vi "LMS_SetupStream.vi"(8 "error in (no error)":errorcluster, 10 "stream_In":T1, 11 "device_In":i64) -> (0 "error out":errorcluster, 1 "steam_Out":T1, 3 "device_Out":i64)   [LabVIEW 2013, in "LMS_LV_Drv.lvlib"]
uses:
  LMS_LV_Drv.lvlib
  Stream_ctl.ctl
  LimeSuite.dll
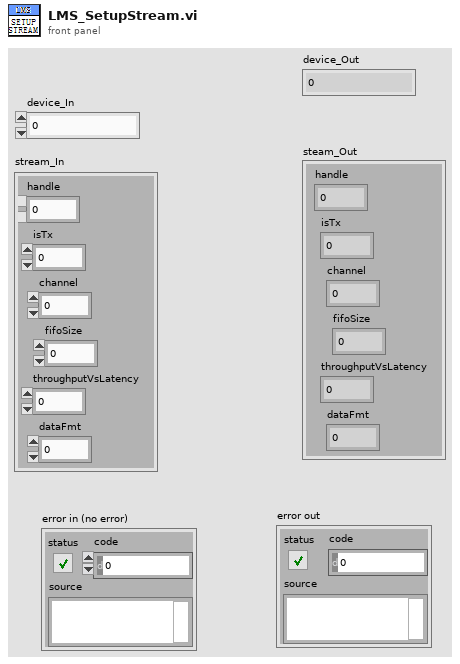
[diagram p1: front panel]
types:
  T1 = typedef "Stream_ctl.ctl" = cluster{"handle":u64, "isTx":u8, "channel":u32, "fifoSize":u32, "throughputVsLatency":dbl, "dataFmt":u32}
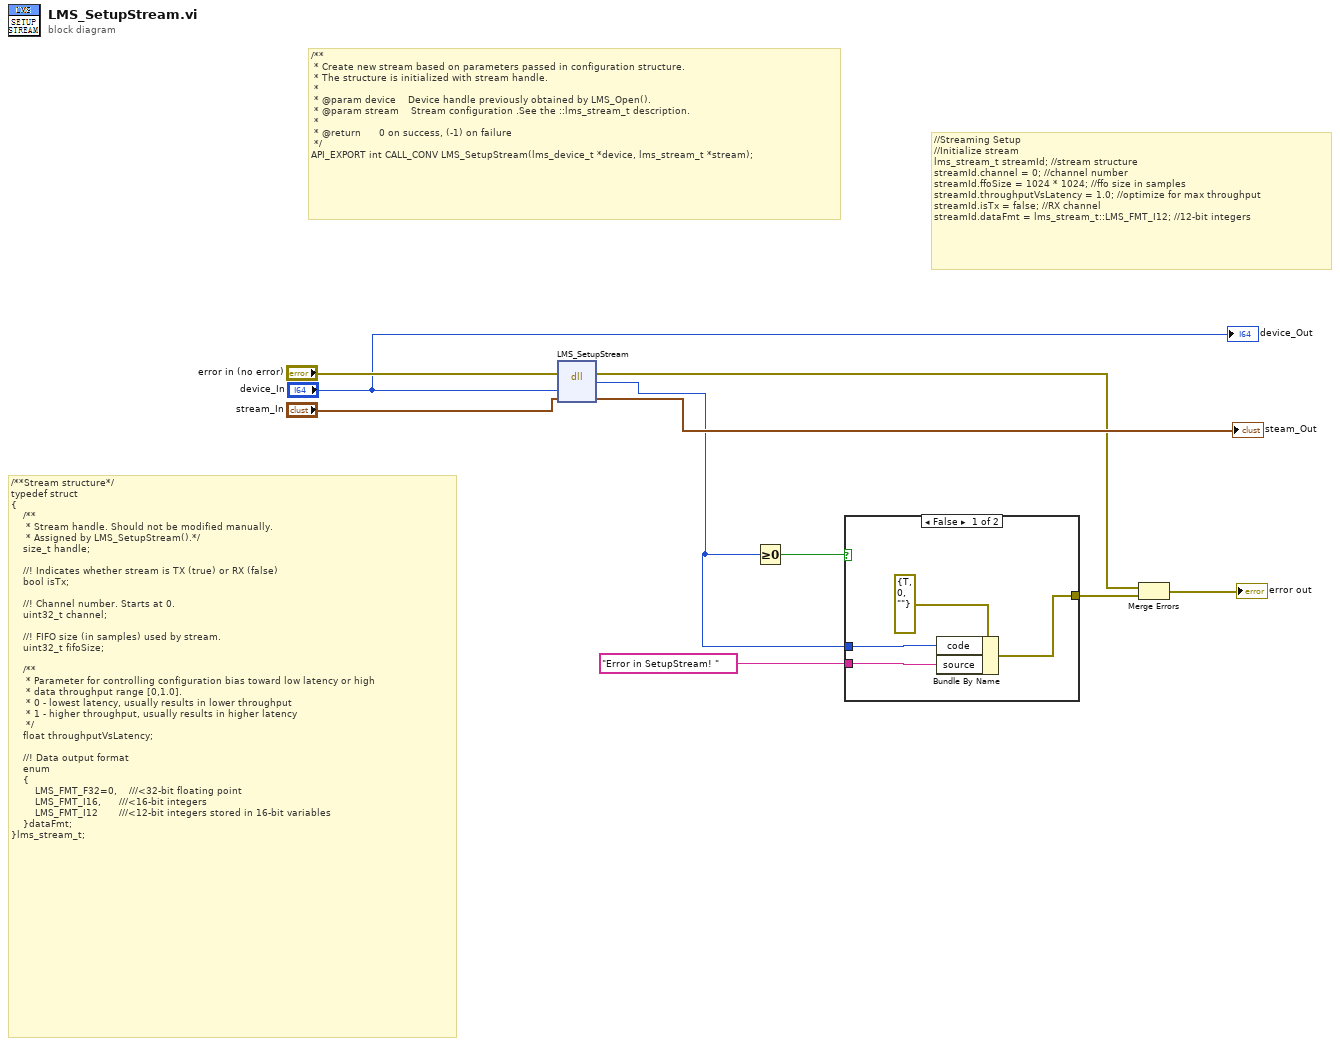
[diagram p0: block diagram]
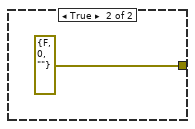
[diagram p2: hidden frame]
diagram:
  # "/**Stream structure*/\ntypedef struct\n{\n    /**\n     * Stream handle. Should not be modified manually.\n     * Assigned by LMS_SetupStream().*/\n    size_t handle;\n\n    //! Indicates whether stream is TX (true) or RX (false)\n    bool isTx;\n\n    //! Channel number. Starts at 0.\n    uint32_t channel;\n\n    //! FIFO size (in samples) used by stream.\n    uint32_t fifoSize;\n\n    /**\n     * Parameter for controlling configuration bias toward low latency or high\n     * data throughput range [0,1.0].\n     * 0 - lowest latency, usually results in lower throughput\n     * 1 - higher throughput, usually results in higher latency\n     */\n    float throughputVsLatency;\n\n    //! Data output format\n    enum\n    {\n        LMS_FMT_F32=0,    ///<32-bit floating point\n        LMS_FMT_I16,      ///<16-bit integers\n        LMS_FMT_I12       ///<12-bit integers stored in 16-bit variables\n    }dataFmt;\n}lms_stream_t;"
  # "//Streaming Setup\n//Initialize stream\nlms_stream_t streamId; //stream structure\nstreamId.channel = 0; //channel number\nstreamId.ffoSize = 1024 * 1024; //ffo size in samples\nstreamId.throughputVsLatency = 1.0; //optimize for max throughput\nstreamId.isTx = false; //RX channel\nstreamId.dataFmt = lms_stream_t::LMS_FMT_I12; //12-bit integers"
  # "/**\n * Create new stream based on parameters passed in configuration structure.\n * The structure is initialized with stream handle.\n *\n * @param device    Device handle previously obtained by LMS_Open().\n * @param stream    Stream configuration .See the ::lms_stream_t description.\n *\n * @return      0 on success, (-1) on failure\n */\nAPI_EXPORT int CALL_CONV LMS_SetupStream(lms_device_t *device, lms_stream_t *stream);"
  n1 = dll-call lib="PTH1mabs CUsersOTADesktop书籍出版程序8.第八章LimeSDR_LabVIEW_Driver-master\nLimeSuite.dll" fn="LMS_SetupStream"(error in="error in (no error)", "device"="device_In", "steam"="stream_In") -> (error out=w2:errorcluster, "return type"=w3:i32, "steam"=→"steam_Out":T1)  [unwired: 3 in, 1 out]
  n2 = Greater Or Equal To 0?(x=w3) -> (x >= 0?=w6:bool)
  n3 = case shown="False" w6 {
    tunnel: [w13 errorcluster {"status"=FALSE, "code"=0, "source"=""} ("error in")] -> w4
    tunnel: w3 -> [w12 _]
    tunnel: "Error in SetupStream! " ("source") -> [w11 _]
    frame False {
      n4 = Bundle By Name(cluster=errorcluster {"status"=TRUE, "code"=0, "source"=""} ("error in"), "code"=w12, "source"=w11) -> (w13:errorcluster)
    }
    frame True {
    }
  }
  n5 = Merge Errors(w2, w4) -> (→"error out":errorcluster)
  "device_Out" <- "device_In"
